vi "Example Callback.vi"() -> ()   [LabVIEW 2013]
uses:
  C:/tf/play/labview/Tinkerforge.dll
panel:
  out "tilt state":string
  in  "stop":bool
  in  "uid":string="gfdd"
  in  "port":i32=4223
  in  "host":string="localhost"
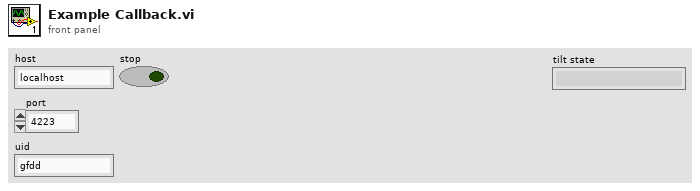
[diagram p1: front panel]
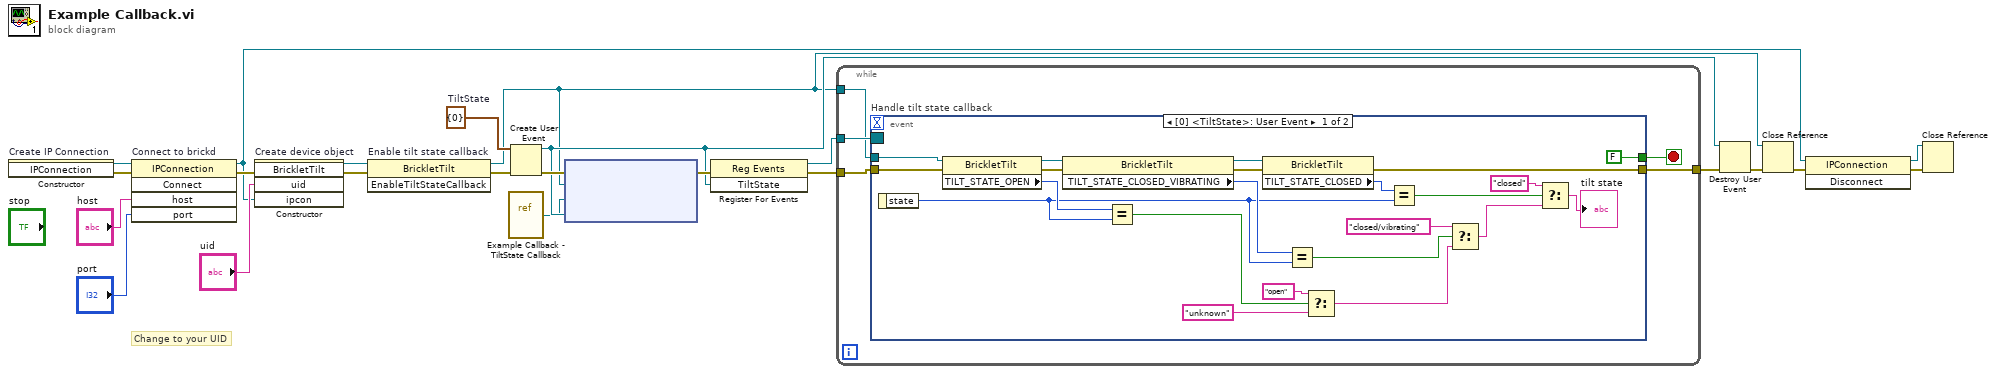
[diagram p0: block diagram]
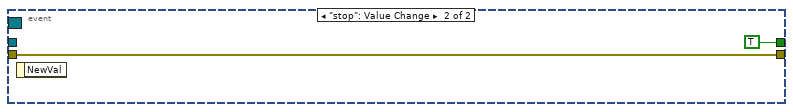
[diagram p2: hidden frame]
diagram:
  w7 = cluster{"state":u8} {"state"=0}  # TiltState
  # "Change to your UID"
  n1 = constructor on="Create IP Connection" class="IPConnection"() -> (reference out=w23:refnum<k24>, error out=w3:errorcluster)  [unwired: 3 in, 1 out]
  n2 = invoke on="Connect to brickd" class="IPConnection" method="Connect"(reference=w23, error in=w3, "host"="host", "port"="port") -> (reference out=w16:refnum<k24>, error out=w19:errorcluster)  [unwired: 1 in, 3 out]
  n3 = constructor on="Create device object" class="BrickletTilt"(error in=w19, "uid"="uid", "ipcon"=w16) -> (reference out=w4:refnum<k24>, error out=w6:errorcluster)  [unwired: 2 in, 3 out]
  n4 = invoke on="Enable tilt state callback" class="BrickletTilt" method="EnableTiltStateCallback"(reference=w4, error in=w6) -> (reference out=w1:refnum<k24>, error out=w5:errorcluster)  [unwired: 1 in, 1 out]
  n5 = vi-ref "Example Callback - TiltState Callback.vi"() -> ("vi reference"=w2:refnum<vi>)
  n6 = Create User Event(user event datatype=w7, error in=w5) -> (user event=w9:refnum<user-event>, error out=w14:errorcluster)
  n7 = node ("Register Event Callback")(w14, w1, w2, w9) -> (w13:errorcluster)  [unwired: 1 in, 1 out]
  n8 = register-events(error in=w13, w9) -> (reference out=w12:refnum<event-registration>, error out=w10:errorcluster)  [unwired: 1 in]
  n9 = while {
    tunnel: w12 -> [w28]
    tunnel: [w27] -> w11
    tunnel: w10 -> [w26]
    tunnel: w1 -> [w24]
    stop <- w25 stop-if-true
    n10 = event "Handle tilt state callback" shown="[0] <TiltState>: User Event" {
      selector: w28 -> [_ _]
      dyn-events: _ -> [_ _]
      timeout: _ -> [_ _]
      tunnel: [w49 w51] -> w27
      tunnel: w26 -> [w35 w51]
      tunnel: [FALSE TRUE] -> w25
      tunnel: w24 -> [w38 _]
      event User Event {
        n11 = event-data() -> ("state"=w33:u8)  [unwired: 1 in]
        n12 = property class="BrickletTilt"(reference=w38, error in=w35) -> (reference out=w37:refnum<k24>, error out=w36:errorcluster, "TILT_STATE_OPEN"=w34:u8)
        n13 = property class="BrickletTilt"(reference=w37, error in=w36) -> (reference out=w44:refnum<k24>, error out=w43:errorcluster, "TILT_STATE_CLOSED_VIBRATING"=w40:u8)
        n14 = Equal?(x=w34, y=w33) -> (x = y?=w32:bool)
        n15 = property class="BrickletTilt"(reference=w44, error in=w43) -> (error out=w49:errorcluster, "TILT_STATE_CLOSED"=w48:u8)  [unwired: 1 out]
        n16 = Equal?(x=w40, y=w33) -> (x = y?=w42:bool)
        n17 = Select(t="open", s=w32, f="unknown") -> (s? t:f=w29:string)
        n18 = Equal?(x=w48, y=w33) -> (x = y?=w47:bool)
        n19 = Select(t="closed/vibrating", s=w42, f=w29) -> (s? t:f=w39:string)
        n20 = Select(t="closed", s=w47, f=w39) -> (s? t:f=→"tilt state":string)
      }
      event "stop": Value Change {
        n21 = event-data() -> ()  [unwired: 1 in, 1 out]
      }
    }
  }
  n22 = Destroy User Event(user event=w9, error in=w11) -> (error out=w8:errorcluster)
  n23 = Close Reference(reference=w1, error in (no error)=w8) -> (error out=w18:errorcluster)
  n24 = invoke class="IPConnection" method="Disconnect"(reference=w16, error in=w18) -> (reference out=w15:refnum<k24>, error out=w17:errorcluster)  [unwired: 1 in, 1 out]
  n25 = Close Reference(reference=w15, error in (no error)=w17) -> ()  [unwired: 1 out]
